vi "integrate test.vi"() -> ()   [LabVIEW 2020]
uses:
  <vilib>/Analysis/3filter.llb/Filter Passband Type.ctl
  <vilib>/Analysis/baseanly.llb/Mean (DBL).vi
  <vilib>/Analysis/3filter.llb/Butterworth Filter (DBL).vi
  <vilib>/Analysis/NI_AALBase.lvlib
panel:
  out "original":cluster{"f0":dbl, "df":dbl, "magnitude":dbl[]}(graph)
  out "cutoff":cluster{"f0":dbl, "df":dbl, "magnitude":dbl[]}(graph)
  in  "high cutoff freq":dbl=30.0 format="%#_13g"
  out "XY Graph 2":cluster{dbl[], "Amplitudes":dbl[]}[](graph)
  out "csapásszám":dbl format="%0.2f"
  in  "low cutoff freq: fl":dbl=30.0 format="%#_13g"
  in  "order":i32=4
  out "original":waveform(dbl)(graph)
  out "mean":dbl format="%0.2f"
  out "cutoff":waveform(dbl)(graph)
  out "XY Graph":cluster{"Ramp Pattern":dbl[], dbl[]}(graph)
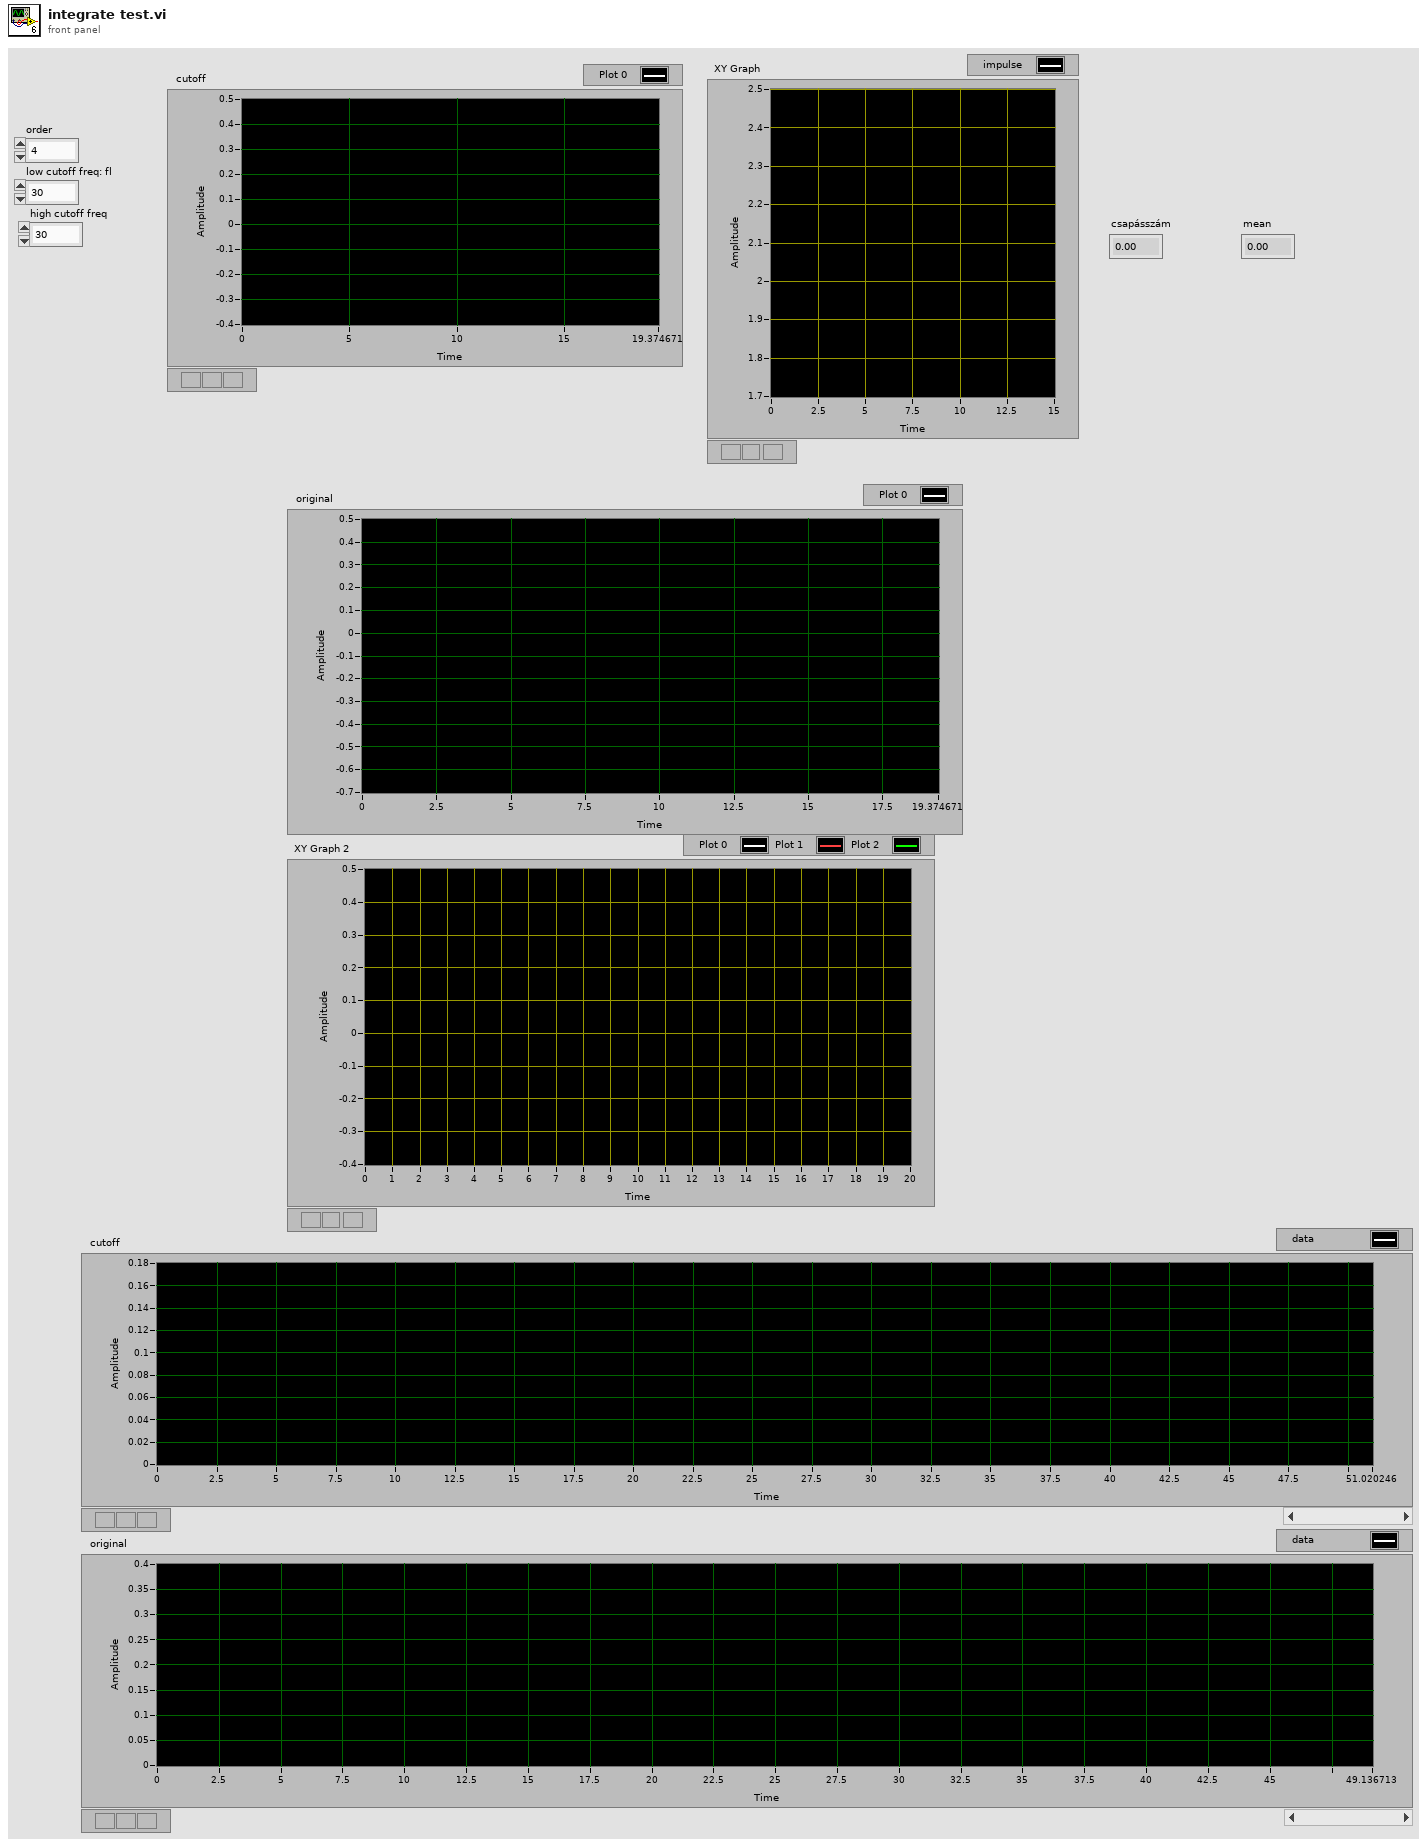
[diagram p1: front panel]
types:
  T1 = typedef "NI_AALBase.lvlib/Filter Passband Type.ctl" = enum32{"Lowpass", "Highpass", "Bandpass", "Bandstop"}
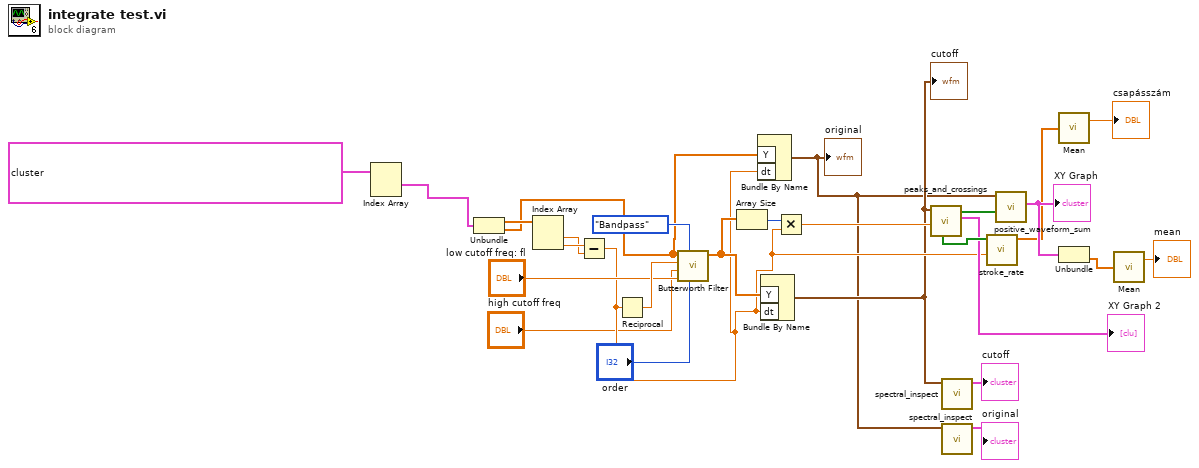
[diagram p0: block diagram]
diagram:
  n1 = Index Array(array=cluster{dbl[], "Amplitudes":dbl[]}[] [{array[2043 elements], "Amplitudes"=array[1980 elements]}, {[1.5763806099757023, 2.8788752707419545, 4.1323493646888405, 5.473433374063183, 6.785512359724196, 7.9462093295011895, 9.166681737720152, 10.53363423723116, 11.756144130324873, 13.061718003611569, 14.263142573740256, 15.551977015208628, 16.803183914022057, 18.17217343692978], "Amplitudes"=[0.4209723817679872, 0.43838008661455447, 0.40969423560903173, 0.42807415249786834, 0.4369954254245966, 0.42537787499984897, 0.38373816002828354, 0.4326666588608348, 0.4094702315237624, 0.41433301820029034, 0.3973110721395309, 0.41324887243155656, 0.3982685319125561, 0.3890943619066075]}, {[0.6069881910078274, 1.2139763820156548, 1.918865894153777, 2.330051442901015, 3.2111633330736677, 3.6419291460469645, 4.493670639880529, 4.944016717079885, 5.805548343026478, 6.187363495434628, 7.058685253494251, 7.499241198580577, 8.350982692414142, 8.76216824116138, 9.69223079189918, 10.025095283742182, 10.857256513349688, 11.248861797870866, 12.0908131595914, 12.590109897355905, 13.392900730624321, 13.833456675710648, 14.646037641092095, 15.027852793500244, 15.928544947898954, 16.339730496646194, 17.201262122592787, 17.769089785148495, 18.562090486303884, 18.953695770825064], "Amplitudes"=[0.0, 0.0, 0.0, 0.0, 0.0, 0.0, 0.0, 0.0, 0.0, 0.0, 0.0, 0.0, 0.0, 0.0, 0.0, 0.0, 0.0, 0.0, 0.0, 0.0, 0.0, 0.0, 0.0, 0.0, 0.0, 0.0, 0.0, 0.0, 0.0, 0.0]}] ("all in array")) -> (element #1=w21:cluster{dbl[], "Amplitudes":dbl[]})  [unwired: 2 in, 1 out]
  n2 = Unbundle(w21) -> (w20:dbl[], "Amplitudes"=w6:dbl[])
  n3 = Index Array(array=w20) -> (element #1=w18:dbl, element #2=w19:dbl)  [unwired: 2 in]
  n4 = Subtract(x=w19, y=w18) -> (x-y=w7:dbl)
  n5 = Reciprocal(x=w7) -> (1/x=w17:dbl)
  n6 = call-poly <vilib>:"Butterworth Filter.vi"("order"="order", "filter type"=Filter_Passband_Type."Bandpass", "low cutoff freq: fl"="low cutoff freq: fl", "high cutoff freq: fh"="high cutoff freq", "sampling freq: fs"=w17, "X"=w6) -> ("Filtered X"=w14:dbl[])  [unwired: 2 in, 1 out]
  n7 = Array Size(array=w14) -> (size(s)=w13:i32)
  n8 = Bundle By Name("Y"=w6, "dt"=w7) -> (w3:waveform(dbl))  [unwired: 1 in]
  "original" <- w3
  n9 = Bundle By Name("Y"=w14, "dt"=w7) -> (w4:waveform(dbl))  [unwired: 1 in]
  "cutoff" <- w4
  n10 = Multiply(x=w13, y=w7) -> (x*y=w12:dbl)
  n11 = call "peaks_and_crossings.vi"("end"=w12, "waveform"=w4) -> ("all in array"=→"XY Graph 2":cluster{dbl[], "Amplitudes":dbl[]}[], "plus-minus crossing?"=w24:bool[], "minus-plus crossing?"=w11:bool[])  [unwired: 3 in, 4 out]
  n12 = call "spectral_inspect.vi"("waveform"=w4) -> ("PSD"=→"cutoff":cluster{"f0":dbl, "df":dbl, "magnitude":dbl[]})  [unwired: 6 in, 4 out]
  n13 = call "spectral_inspect.vi"("waveform"=w3) -> ("PSD"=→"original":cluster{"f0":dbl, "df":dbl, "magnitude":dbl[]})  [unwired: 6 in, 4 out]
  n14 = call "stroke_rate.vi"("dt"=w7, "minus-plus"=w11) -> ("stroke rate"=w10:dbl[])  [unwired: 9 in]
  n15 = call "positive_waveform_sum.vi"("plus-minus"=w24, "read in data"=w3) -> ("csapás impulzus"=w27:cluster{"Ramp Pattern":dbl[], dbl[]})  [unwired: 8 in, 1 out]
  "XY Graph" <- w27
  n16 = call-poly <vilib>:"Mean.vi"("X"=w10) -> ("mean"=→"csapásszám":dbl)  [unwired: 1 out]
  n17 = Unbundle(w27) -> (w26:dbl[])  [unwired: 1 out]
  n18 = call-poly <vilib>:"Mean.vi"("X"=w26) -> ("mean"=→"mean":dbl)  [unwired: 1 out]
